vi "rectangleCheck0.vi"(11 "rectangle":cluster{"x1":i32, "y1":i32, "x2":i32, "y2":i32}) -> (3 "rectangle out":cluster{"x1":i32, "y1":i32})   [LabVIEW 2011]
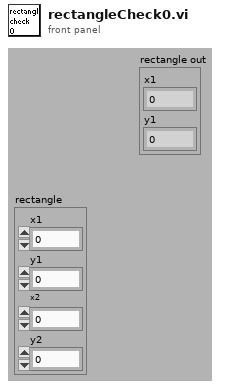
[diagram p1: front panel]
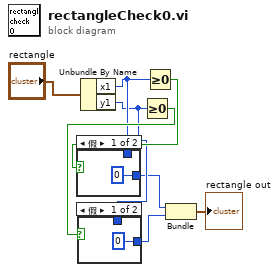
[diagram p0: block diagram]
diagram:
  n1 = Unbundle By Name("rectangle") -> ("x1"=w5:i32, "y1"=w4:i32)
  n2 = Greater Or Equal To 0?(x=w4) -> (x >= 0?=w6:bool)
  n3 = case shown="假" w6 {
    tunnel: [0 ("y1") w10] -> w3
    tunnel: w4 -> [_ w10]
    frame False {
    }
    frame True {
    }
  }
  n4 = Greater Or Equal To 0?(x=w5) -> (x >= 0?=w7:bool)
  n5 = case shown="假" w7 {
    tunnel: [0 ("x1") w12] -> w2
    tunnel: w5 -> [_ w12]
    frame False {
    }
    frame True {
    }
  }
  n6 = Bundle("x1"=w2, "y1"=w3) -> (→"rectangle out":cluster{"x1":i32, "y1":i32})  [unwired: 1 out]
